vi "toml.vi"() -> ()   [LabVIEW 2020]
uses:
  dragon_toml_64.dll
panel:
  in  "subkey (optional)":string="version"
  in  "subtable_name (optional)":string="dependencies"
  in  "file_path":path=path "Y:/JKI/GitHub/labview-project-load-tools/rust_src/toml_edit_dll/lv_src/test.toml"
  out "result":i32
  out "error out":errorcluster={"status"=TRUE, "code"=1097, "source"="Call Library Function Node in toml.vi"}
  in  "value":string="1.2.3"
  in  "key_name":string="my_package"
  in  "table_name":string="nipm"
  in  "error in (no error)":errorcluster
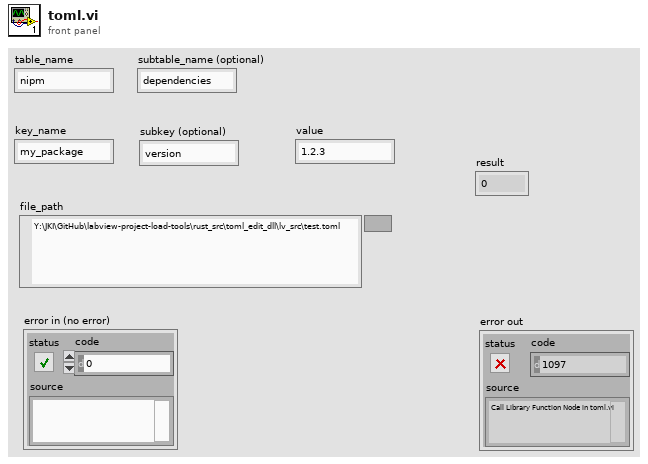
[diagram p1: front panel]
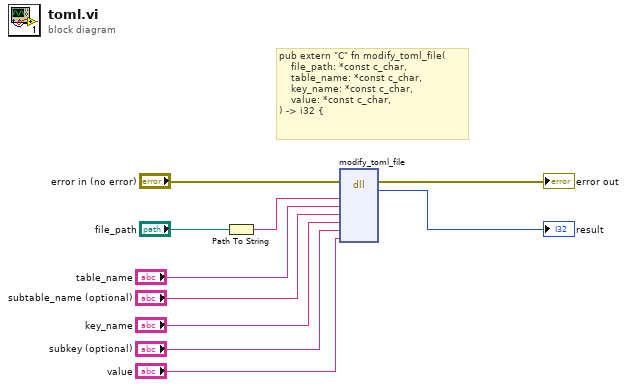
[diagram p0: block diagram]
diagram:
  # "pub extern \"C\" fn modify_toml_file(\n    file_path: *const c_char,\n    table_name: *const c_char,\n    key_name: *const c_char,\n    value: *const c_char,\n) -> i32 {"
  n1 = Path To String(path="file_path") -> (string=w3:string)
  n2 = dll-call lib="C:/Projects/labview-project-load-tools/rust_src/toml_edit_dll/lv_src/dragon_toml**.dll" fn="modify_toml_file"(error in="error in (no error)", "file_path"=w3, "table_name"="table_name", "subtable_name"="subtable_name (optional)", "key_name"="key_name", "subkey_name"="subkey (optional)", "value"="value") -> (error out=→"error out":errorcluster, "result"=→"result":i32)  [unwired: 8 in, 1 out]
